vi "File.Filter Path By Name.vi"(9 "Order By Filter":bool, 10 "Filter1":string[](array[string]), 11 "Paths":path[](array[path])) -> (3 "Paths Out":path[](array[path]))   [LabVIEW 2024]
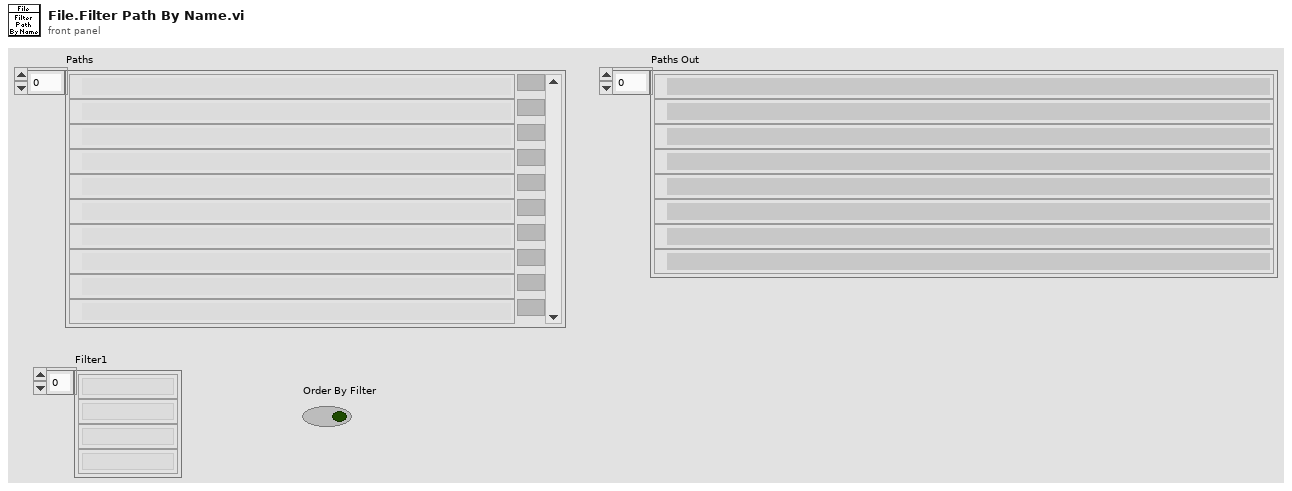
[diagram p1: front panel]
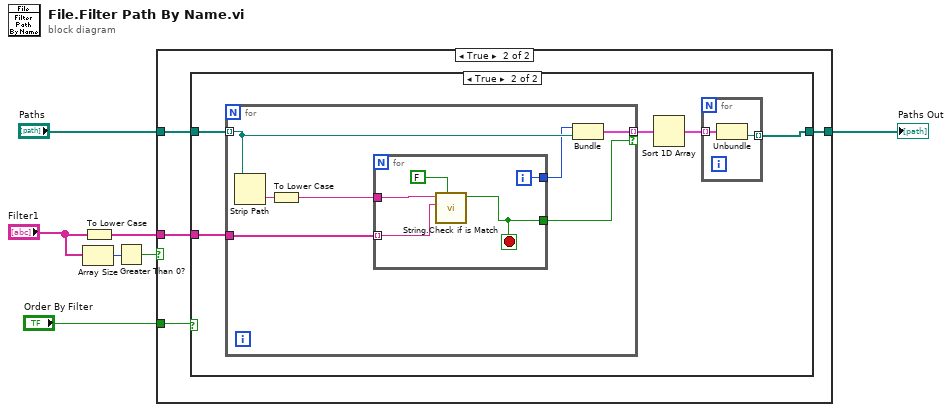
[diagram p0: block diagram]
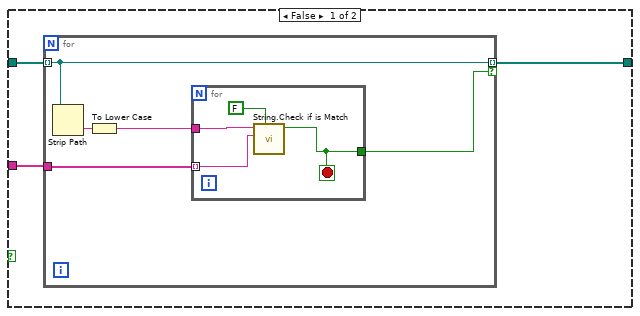
[diagram p3: hidden frame]
diagram:
  n1 = Array Size(array="Filter1") -> (size(s)=w6:i32)
  n2 = To Lower Case(string="Filter1") -> (all lower case string=w3:string[])
  n3 = Greater Than 0?(x=w6) -> (x > 0?=w5:bool)
  n4 = case shown="True" w5 {
    tunnel: "Paths" -> [w8 w12]
    tunnel: w3 -> [_ w11]
    tunnel: [w8 w10] -> w2
    tunnel: "Order By Filter" -> [_ w9]
    frame False {
    }
    frame True {
      n5 = case shown="True" w9 {
        tunnel: w12 -> [w15 w29]
        tunnel: w11 -> [w14 w28]
        tunnel: [w13 w25] -> w10
        frame False {
          n6 = for {
            tunnel: w15 -> [w20] mode=indexing
            tunnel: w14 -> [w19]
            tunnel: [w20] -> w13 mode=indexing if=w16
            n7 = Strip Path(path=w20) -> (name=w18:string)  [unwired: 1 out]
            n8 = To Lower Case(string=w18) -> (all lower case string=w17:string)
            n9 = for {
              tunnel: w17 -> [w24]
              tunnel: w19 -> [w23] mode=indexing
              tunnel: [w22] -> w16
              stop <- w22 stop-if-true
              n10 = call "String.Check if is Match.vi"("And(F)/Or(T)"=FALSE, "CSV Pattern List"=w23, "String"=w24) -> ("Is Match"=w22:bool)  [unwired: 8 in]
            }
          }
        }
        frame True {
          n11 = for {
            tunnel: w29 -> [w34] mode=indexing
            tunnel: w28 -> [w38]
            tunnel: [w33] -> w27 mode=indexing if=w35
            n12 = Strip Path(path=w34) -> (name=w37:string)  [unwired: 1 out]
            n13 = To Lower Case(string=w37) -> (all lower case string=w36:string)
            n14 = for {
              tunnel: w36 -> [w43]
              tunnel: w38 -> [w42] mode=indexing
              tunnel: [w41] -> w35
              tunnel: [w39] -> w32
              i -> [w39]
              stop <- w41 stop-if-true
              n15 = call "String.Check if is Match.vi"("And(F)/Or(T)"=FALSE, "CSV Pattern List"=w42, "String"=w43) -> ("Is Match"=w41:bool)  [unwired: 8 in]
            }
            n16 = Bundle(w32, "Path"=w34) -> (w33:cluster{i32, "Path":path})  [unwired: 1 in]
          }
          n17 = Sort 1D Array(array=w27) -> (sorted array=w26:cluster{i32, "Path":path}[])
          n18 = for {
            tunnel: w26 -> [w31] mode=indexing
            tunnel: [w30] -> w25 mode=indexing
            n19 = Unbundle(w31) -> ("Path"=w30:path)  [unwired: 1 out]
          }
        }
      }
    }
  }
  "Paths Out" <- w2
